vi "Shoot.vi"(2 "Reset":bool, 3 "Safety Override":bool, 5 "Shoot":bool) -> (0 "State":T1(ring), 1 "Finished Cycle":bool)   [LabVIEW 2013]
doc: "Shoots a ball. \nShoot is a boolean input that needs only to be pulsed, and then the entire automated shooting sequence will be run. The shooter normally only fires when a ball is detected, but you can override this by wiring a boolean to Safety Override. Reset is an input which aborts the shooting cycle. Finished Cycle is an output which pulses True once the ball has been fired and the shooter has been reset. State is an Enum which describes the state of the shooting sequence. Look at the state machine in this VI to see what these states are."
uses:
  <vilib>/Rock Robotics/WPI/Solenoid/WPI_SolenoidValue.ctl
  <vilib>/Rock Robotics/WPI/Solenoid/WPI_SolenoidSetEnum.vi
  <vilib>/Rock Robotics/WPI/Solenoid/WPI_SolenoidGetEnum.vi
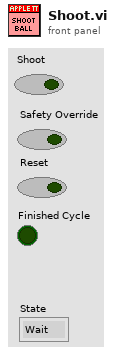
[diagram p1: front panel]
types:
  T1 = enum16{"Wait", "Clear", "Release", "Cock", "Reset"}
  T2 = typedef "WPI_SolenoidDevRef.ctl" = cluster{"DevStatus":errorcluster, "Solenoid Module":T3, "Forward Solenoid Channel":T4, "Reverse Solenoid Channel":T4}
  T3 = typedef "FPGA_TypedefSolenoidModule.ctl" = enum16{"Solenoid Module 1", "Solenoid Module 2"}
  T4 = typedef "WPI_SolenoidChannel.ctl" = enum8{"Solenoid 1", "Solenoid 2", "Solenoid 3", "Solenoid 4", "Solenoid 5", "Solenoid 6", "Solenoid 7", "Solenoid 8", "Invalid"}
  T5 = typedef "WPI_SolenoidValue.ctl" = enum16{"Off", "On", "Forward", "Reverse"}
  T6 = typedef "WPI_MotorControlDeviceRef.ctl" = cluster{"DeviceStatus":errorcluster, "Type":enum16{"PWM", "CAN"}, "PWM":cluster{"Digital Module":T7, "PWM Channel":T8, "DeadBand":T9}, "CAN":cluster{"Device Number":u8, "Control Mode":T10, "Semaphore":T11, "Max Vout":dbl}, "Invert":bool, "TransformRef":T12, "InvTransformRef":T12}
  T7 = typedef "FPGA_TypedefDigitalModule.ctl" = enum16{"Digital Module 1", "Digital Module 2"}
  T8 = typedef "FPGA_DIOPWMChannel.ctl" = enum8{"PWM 1", "PWM 2", "PWM 3", "PWM 4", "PWM 5", "PWM 6", "PWM 7", "PWM 8", "PWM 9", "PWM 10", "Invalid"}
  T9 = typedef "WPI_PWMDeadband.ctl" = cluster{"Name":string, "maxPositivePwm":i32, "minPositivePwm":i32, "centerPwm":i32, "maxNegativePwm":i32, "minNegativePwm":i32, "angularRange":u16}
  T10 = typedef "WPI_CANJaguar_ControlMode.ctl" = enum8{"Percent VBus", "Current", "Speed", "Position", "Voltage"}
  T11 = typedef "Semaphore RefNum" = refnum<k1>
  T12 = typedef "WPI_PWMTransform_ConPane.ctl" = refnum<vi>
  T13 = typedef "WPI_DigitalInputDevRef.ctl" = cluster{"DevStatus":errorcluster, "DIO Channel":T14, "Digital Module":T7}
  T14 = typedef "FPGA_DIOChannel.ctl" = enum8{"DIO 1", "DIO 2", "DIO 3", "DIO 4", "DIO 5", "DIO 6", "DIO 7", "DIO 8", "DIO 9", "DIO 10", "DIO 11", "DIO 12", "DIO 13", "DIO 14", "Invalid"}
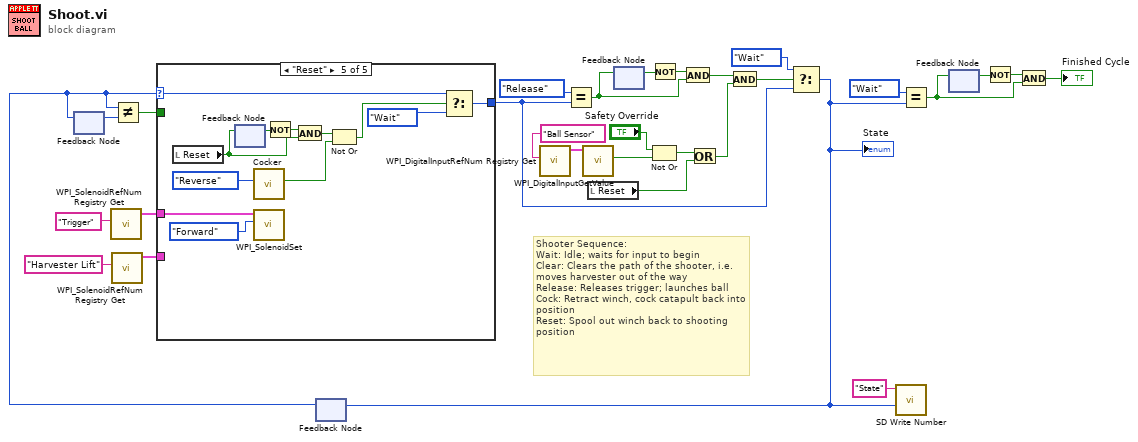
[diagram p0: block diagram]
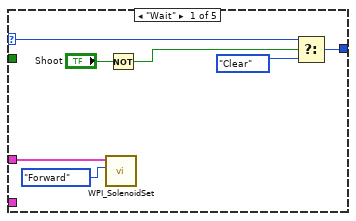
[diagram p2: hidden frame]
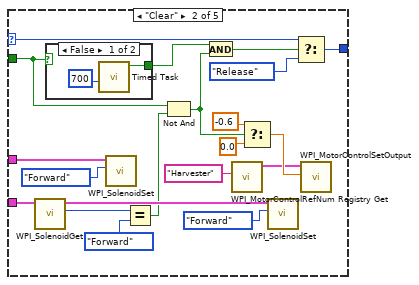
[diagram p3: hidden frame]
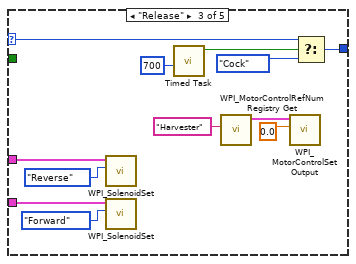
[diagram p5: hidden frame]
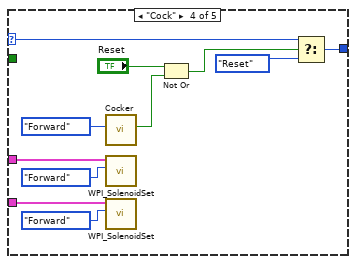
[diagram p6: hidden frame]
diagram:
  # "Shooter Sequence:\nWait: Idle; waits for input to begin\nClear: Clears the path of the shooter, i.e. moves harvester out of the way\nRelease: Releases trigger; launches ball\nCock: Retract winch, cock catapult back into position\nReset: Spool out winch back to shooting position"
  n1 = feedback #1() -> (w21:T1)  [unwired: 1 in]
  n2 = call <vilib>:"WPI_SolenoidRefNum Registry Get.vi"("refnum name"="Trigger") -> ("SolenoidDevRef"=w22:T2)  [unwired: 9 in, 1 out]
  n3 = call <vilib>:"WPI_SolenoidRefNum Registry Get.vi"("refnum name"="Harvester Lift") -> ("SolenoidDevRef"=w27:T2)  [unwired: 9 in, 1 out]
  n4 = feedback #2() -> (w20:T1)  [unwired: 1 in]
  n5 = feedback-in #1(w20) -> ()
  n6 = Not Equal?(x=w20, y=w21) -> (x != y?=w19:bool)
  n7 = case shown="\"Reset\"" w20 {
    selector: w20 -> [w34 w54 w70 w80 w92]
    tunnel: [w33 w55 w71 w81 w93] -> w7
    tunnel: w27 -> [_ w51 w62 w76 _]
    tunnel: w22 -> [w30 w40 w67 w78 w90]
    tunnel: w19 -> [_ w37 _ _ _]
    frame "Wait" {
      n8 = call-poly <vilib>:"WPI_SolenoidSet.vi"("Value"=WPI_SolenoidValue."Forward", "SolenoidDevRef"=w30) -> ()  [unwired: 8 in, 2 out]
      n9 = Not(x="Shoot") -> (.not. x?=w32:bool)
      n10 = Select(t=w34, s=w32, f=T1."Clear") -> (s? t:f=w33:T1)
    }
    frame "Clear" {
      n11 = call-poly <vilib>:"WPI_SolenoidGet.vi"("SolenoidDevRef"=w51) -> ("Value"=w44:T5, "SolenoidDevRef"=w52:T2)  [unwired: 8 in, 1 out]
      n12 = case shown="False" w37 {
        selector: w37 -> [_ w59]
        tunnel: [w57 w59] -> w38
        frame False {
          n13 = call "Timed Task.vi"("Time (ms)"=u32 700) -> ("Running"=w57:bool)  [unwired: 10 in]
        }
        frame True {
        }
      }
      n14 = call-poly <vilib>:"WPI_SolenoidSet.vi"("Value"=WPI_SolenoidValue."Forward", "SolenoidDevRef"=w40) -> ()  [unwired: 8 in, 2 out]
      n15 = Equal?(x=w44, y=WPI_SolenoidValue."Forward" ("Value")) -> (x = y?=w39:bool)
      n16 = Not And(1:w39, 2:w37) -> (0:w43:bool)
      n17 = And(x=w38, y=w43) -> (x .and. y?=w50:bool)
      n18 = call <vilib>:"WPI_MotorControlRefNum Registry Get.vi"("refnum name"="Harvester") -> ("MotorControlDevRef"=w45:T6)  [unwired: 9 in, 1 out]
      n19 = Select(t=-0.6, s=w43, f=0.0) -> (s? t:f=w46:dbl)
      n20 = call-poly <vilib>:"WPI_SolenoidSet.vi"("Value"=WPI_SolenoidValue."Forward", "SolenoidDevRef"=w52) -> ()  [unwired: 8 in, 2 out]
      n21 = Select(t=w54, s=w50, f=T1."Release") -> (s? t:f=w55:T1)
      n22 = call <vilib>:"WPI_MotorControlSetOutput.vi"("Output"=w46, "MotorControlDevRef"=w45) -> ()  [unwired: 7 in, 3 out]
    }
    frame "Release" {
      n23 = call-poly <vilib>:"WPI_SolenoidSet.vi"("Value"=WPI_SolenoidValue."Reverse", "SolenoidDevRef"=w67) -> ()  [unwired: 8 in, 2 out]
      n24 = call-poly <vilib>:"WPI_SolenoidSet.vi"("Value"=WPI_SolenoidValue."Forward", "SolenoidDevRef"=w62) -> ()  [unwired: 8 in, 2 out]
      n25 = call "Timed Task.vi"("Time (ms)"=u32 700) -> ("Running"=w60:bool)  [unwired: 10 in]
      n26 = call <vilib>:"WPI_MotorControlRefNum Registry Get.vi"("refnum name"="Harvester") -> ("MotorControlDevRef"=w65:T6)  [unwired: 9 in, 1 out]
      n27 = call <vilib>:"WPI_MotorControlSetOutput.vi"("Output"=0.0, "MotorControlDevRef"=w65) -> ()  [unwired: 7 in, 3 out]
      n28 = Select(t=w70, s=w60, f=T1."Cock") -> (s? t:f=w71:T1)
    }
    frame "Cock" {
      n29 = call "Cocker.vi"("Position"=enum16{"Forward", "Reverse"}."Forward") -> ("In Position"=w72:bool)  [unwired: 10 in]
      n30 = call-poly <vilib>:"WPI_SolenoidSet.vi"("Value"=WPI_SolenoidValue."Forward", "SolenoidDevRef"=w78) -> ()  [unwired: 8 in, 2 out]
      n31 = call-poly <vilib>:"WPI_SolenoidSet.vi"("Value"=WPI_SolenoidValue."Forward", "SolenoidDevRef"=w76) -> ()  [unwired: 8 in, 2 out]
      n32 = Not Or(1:w72, 2:"Reset") -> (0:w75:bool)
      n33 = Select(t=w80, s=w75, f=T1."Reset") -> (s? t:f=w81:T1)
    }
    frame "Reset" {
      n34 = local read "Reset"() -> (w84:bool)
      n35 = feedback #3() -> (w85:bool)  [unwired: 1 in]
      n36 = feedback-in #3(w84) -> ()
      n37 = call "Cocker.vi"("Position"=enum16{"Forward", "Reverse"}."Reverse") -> ("In Position"=w88:bool)  [unwired: 10 in]
      n38 = call-poly <vilib>:"WPI_SolenoidSet.vi"("Value"=WPI_SolenoidValue."Forward", "SolenoidDevRef"=w90) -> ()  [unwired: 8 in, 2 out]
      n39 = Not(x=w85) -> (.not. x?=w86:bool)
      n40 = And(x=w86, y=w84) -> (x .and. y?=w83:bool)
      n41 = Not Or(1:w88, 2:w83) -> (0:w87:bool)
      n42 = Select(t=w92, s=w87, f=T1."Wait") -> (s? t:f=w93:T1)
    }
  }
  n43 = call <vilib>:"WPI_DigitalInputRefNum Registry Get.vi"("refnum name"="Ball Sensor") -> ("DigitalInputDevRef"=w11:T13)  [unwired: 9 in, 1 out]
  n44 = Equal?(x=T1."Release", y=w7) -> (x = y?=w13:bool)
  n45 = call <vilib>:"WPI_DigitalInputGetValue.vi"("DigitalInputDevRef"=w11) -> ("Value"=w5:bool)  [unwired: 8 in, 2 out]
  n46 = local read "Reset"() -> (w1:bool)
  n47 = feedback #4() -> (w14:bool)  [unwired: 1 in]
  n48 = feedback-in #4(w13) -> ()
  n49 = Not Or(1:w5, 2:"Safety Override") -> (0:w3:bool)
  n50 = Not(x=w14) -> (.not. x?=w15:bool)
  n51 = And(x=w15, y=w13) -> (x .and. y?=w10:bool)
  n52 = Or(x=w3, y=w1) -> (x .or. y?=w2:bool)
  n53 = And(x=w10, y=w2) -> (x .and. y?=w9:bool)
  n54 = Select(t=T1."Wait" ("x"), s=w9, f=w7) -> (s? t:f=w6:T1)
  "State" <- w6
  n55 = feedback-in #2(w6) -> ()
  n56 = call <vilib>:"SD Write Number.vi"("Numeric"=w6, "Name"="State") -> ()  [unwired: 8 in, 2 out]
  n57 = Equal?(x=T1."Wait", y=w6) -> (x = y?=w17:bool)
  n58 = feedback-in #5(w17) -> ()
  n59 = feedback #5() -> (w25:bool)  [unwired: 1 in]
  n60 = Not(x=w25) -> (.not. x?=w24:bool)
  n61 = And(x=w24, y=w17) -> (x .and. y?=→"Finished Cycle":bool)
